vi "Do End Game.vi"(11 "Team in":refnum<class "Team.lvclass">) -> (3 "Team out":refnum<class "Team.lvclass">)   [LabVIEW 2020, in "SquareBattle.lvlib" / "Team.lvclass"]
uses:
  Team.lvclass
  Team Stats.ctl
  Team.lvclass/Team.ctl
  SquareBattle.lvlib
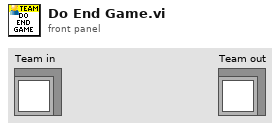
[diagram p1: front panel]
types:
  T1 = typedef "SquareBattle.lvlib/Team Stats.ctl" = cluster{"Active":i32, "Generated":i32, "Kills":i32, "Eliminated":i32, "Collided":i32}
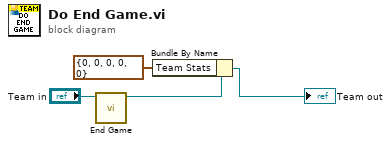
[diagram p0: block diagram]
diagram:
  n1 = call-dynamic "End Game.vi"("Team in"="Team in") -> ("Team out"=w3:refnum<class "Team.lvclass">)  [unwired: 10 in]
  n2 = Bundle By Name(cluster=w3, "Team Stats"=T1 {"Active"=0, "Generated"=0, "Kills"=0, "Eliminated"=0, "Collided"=0}) -> (→"Team out":refnum<class "Team.lvclass">)
